vi "ziExample-Module-DAQ_Spectrum.vi"() -> ()   [LabVIEW 2009]
doc: "Control a Zurich instrument device via the LabOne Labview API. \nRequirements: Zurich Instruments MFLI, HF2 or UHFLI \nThis example shows how to start a spectrum modul and retrieve the Data.\n\n© Zurich Instruments AG, www.zhinst.com"
uses:
  <instrlib>/Zurich Instruments LabOne/Public/Data/ziTypeDoubleDataTS.ctl
  <instrlib>/Zurich Instruments LabOne/Public/Modules/ziTypeModResults.ctl
  <instrlib>/Zurich Instruments LabOne/Public/Data/ziTypePollType.ctl
  <instrlib>/Zurich Instruments LabOne/Public/Modules/ziTypeModGenericHeader.ctl
  <instrlib>/Zurich Instruments LabOne/Public/Modules/ziTypeModEnum.ctl
  <instrlib>/Zurich Instruments LabOne/Public/Modules/ziModSetValueDoubleArray.vi
  <instrlib>/Zurich Instruments LabOne/Public/Modules/ziModSetValueBinary.vi
  <instrlib>/Zurich Instruments LabOne/Public/Configure/ziSetValueDouble.vi
  <instrlib>/Zurich Instruments LabOne/Public/Modules/ziModGetNodeValueDouble.vi
  <instrlib>/Zurich Instruments LabOne/Public/Modules/ziModGetDoubleData.vi
  <instrlib>/Zurich Instruments LabOne/Zurich Instruments LabOne.lvlib
panel:
  out "Finished":bool
  out "Duration":dbl caption="Duration (s)"
  out "Progress (unity)":dbl(slide) step=1.10684602706915e-310 scale=0.0..100.0
  out "Filter":T1[](array[typedef])
  out "Header":T2
  out "Spectrum":T1[](array[typedef])
  in  "subscribepath":string="demods/0/sample.XiY.fft.abs.avg"
  in  "start_act":bool
  in  "stop":bool
  out "Error Out":errorcluster
  out "Power":bool
  out "SpectrumAbs":cluster{dbl[], "Value":dbl[]}[](graph)
  in  "refreshrate":dbl=5.0
  in  "frequencyspan":dbl=13000.0
  in  "Window":u16(ring) items=["Rectangular", "Hann", "Hamming", "Blackman Harris"]
  in  "Absolute":bool
  in  "specdens":bool caption="Spectral Density"
  in  "filtcomp":bool caption="Filter Compensation"
  in  "Address":string="DEV"
  out "Selected Device":string
  # "ziExample-Module-DAQ_Spectrum.vi\nRequirements: HF2LI, UHFLI or MFLI\nsee block diagram for VI description"
  # "Tested Devices:\n- HF2LI\n- UHFLI\n- MFLI"
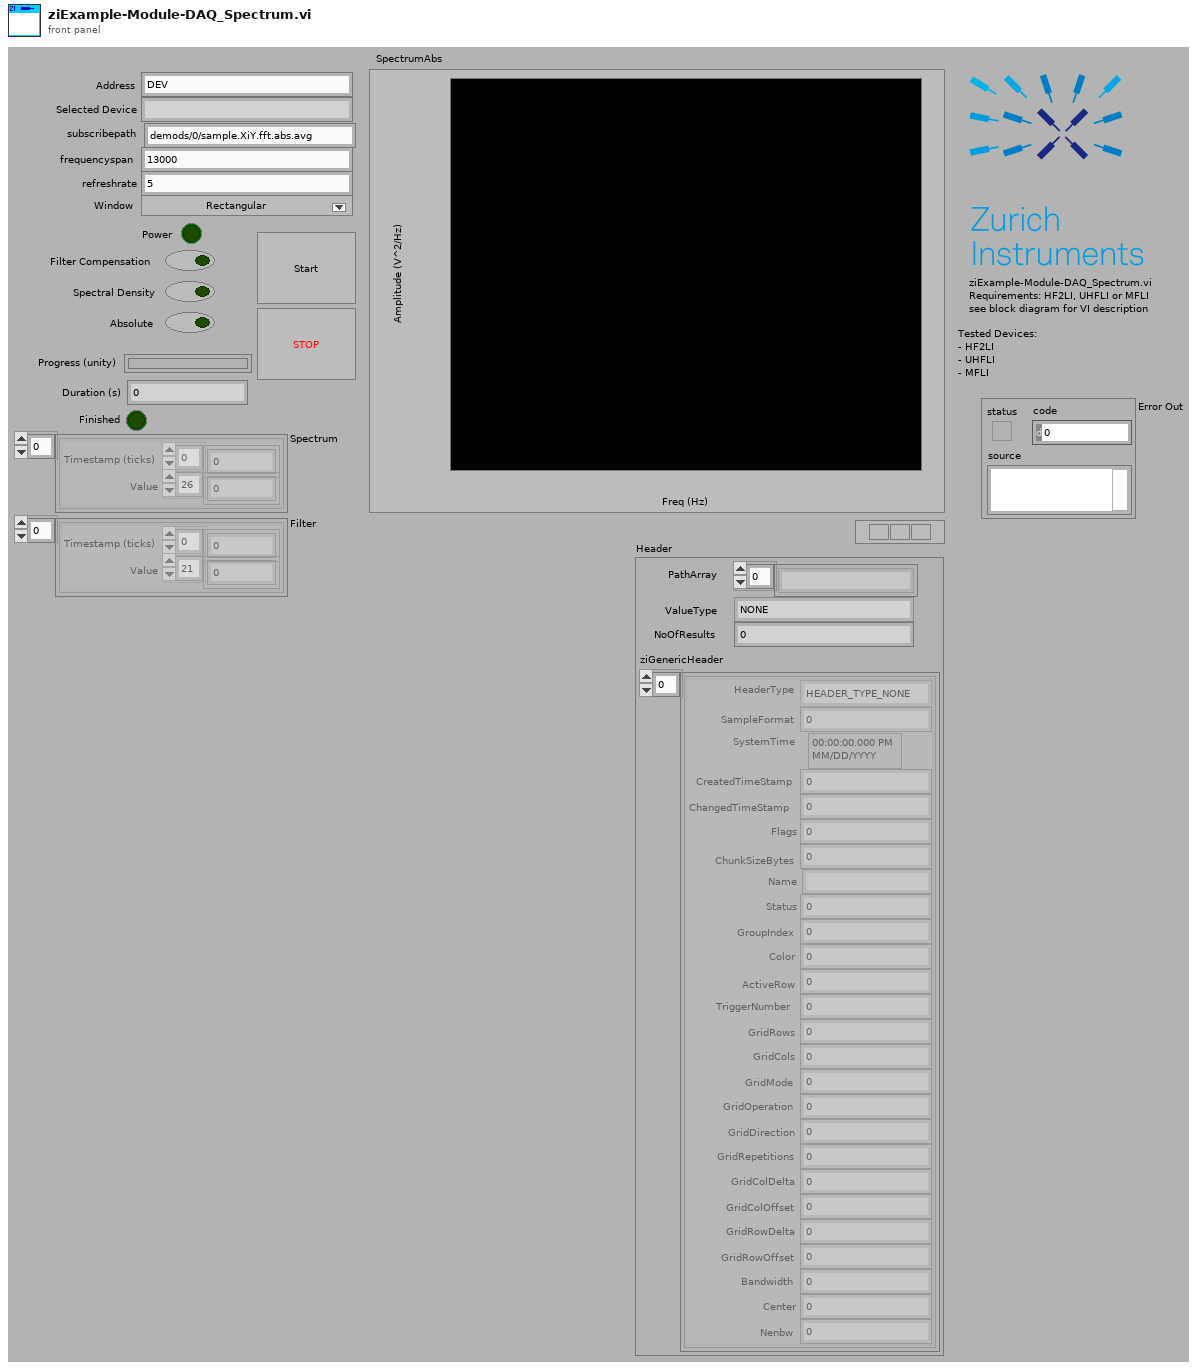
[diagram p1: front panel]
types:
  T1 = typedef "Zurich Instruments LabOne.lvlib/ziTypeDoubleDataTS.ctl" = cluster{"Timestamp (ticks)":u64[], "Value":dbl[]}
  T2 = typedef "Zurich Instruments LabOne.lvlib/ziTypeModResults.ctl" = cluster{"PathArray":string[], "ValueType":T3, "NoOfResults":u64, "ziGenericHeader":T4[]}
  T3 = typedef "Zurich Instruments LabOne.lvlib/ziTypePollType.ctl" = enum16{"NONE", "DOUBLE_DATA", "INTEGER_DATA", "DEMOD_SAMPLE", "SCOPE_WAVE_HF2", "AUXIN_SAMPLE", "DIO_SAMPLE", "BYTE_ARRAY", "PWA_WAVE", "9", "10", "11", "12", "13", "14", "15", "TREE_CHANGE_DEPRI", "17", "ERROR", "19", "20", "21", "22", "23", "24", "25", "26", "27", "28", "29", "30", "31", "DOUBLE_DATA_TS", "INTEGER_DATA_TS", "34", "SCOPE_WAVE", "SCOPE_WAVE_EX", "37", "BYTE_ARRAY_TS", "39", "40", "41", "42", "43", "44", "45", "CNT_DATA", "47", "TREE_CHANGE", "49", "50", "51", "52", "53", "54", "55", "56", "57", "58", "59", "60", "61", "62", "63", "SWEEPER_DATA", "SPECTRUM_DATA", "ADVISOR_DATA", "VECTOR_DATA", "IMP_DATA"}
  T4 = typedef "Zurich Instruments LabOne.lvlib/ziTypeModGenericHeader.ctl" = cluster{"HeaderType":enum8{"HEADER_TYPE_NONE", "HEADER_TYPE_SWTRIGGER", "HEADER_TYPE_SWEEPER"}, "SampleFormat":u8, "SystemTime":timestamp, "CreatedTimeStamp":u64, "ChangedTimeStamp":u64, "Flags":u32, "ChunkSizeBytes":u64, "Name":string, "Status":u32, "GroupIndex":u32, "Color":u32, "ActiveRow":u32, "TriggerNumber":u64, "GridRows":u32, "GridCols":u32, "GridMode":u32, "GridOperation":u32, "GridDirection":u32, "GridRepetitions":u32, "GridColDelta":dbl, "GridColOffset":dbl, "GridRowDelta":dbl, "GridRowOffset":dbl, "Bandwidth":dbl, "Center":dbl, "Nenbw":dbl}
  T5 = typedef "Zurich Instruments LabOne.lvlib/ziTypeModEnum.ctl" = u16
  T6 = typedef "Zurich Instruments LabOne.lvlib/ziTypeHandle.ctl" = cluster{"handleValid":bool, "Conn":u64, "Path Prefix":string, "Handle":u64, "Connected":bool, "Clockbase(s)":dbl}
  T7 = typedef "Zurich Instruments LabOne.lvlib/ziTypeModHandle.ctl" = cluster{"handleValid":bool, "Conn":u64, "ModHandle":u64, "moduleID":string, "Path Prefix":string}
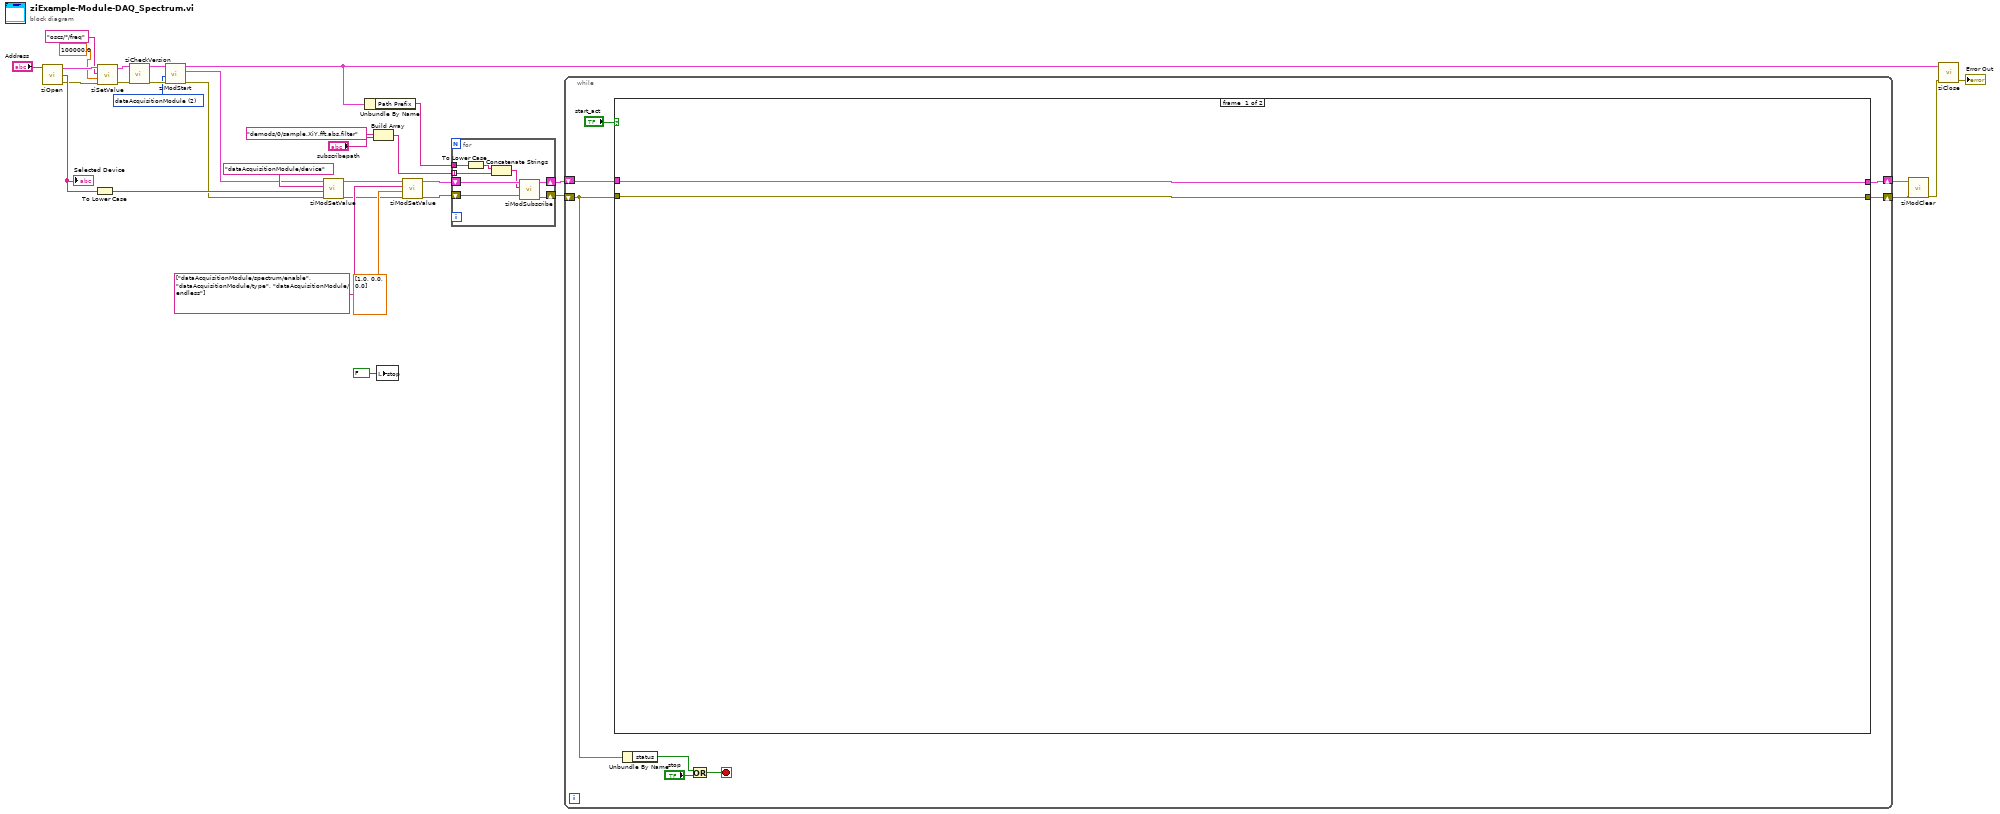
[diagram p0: block diagram]
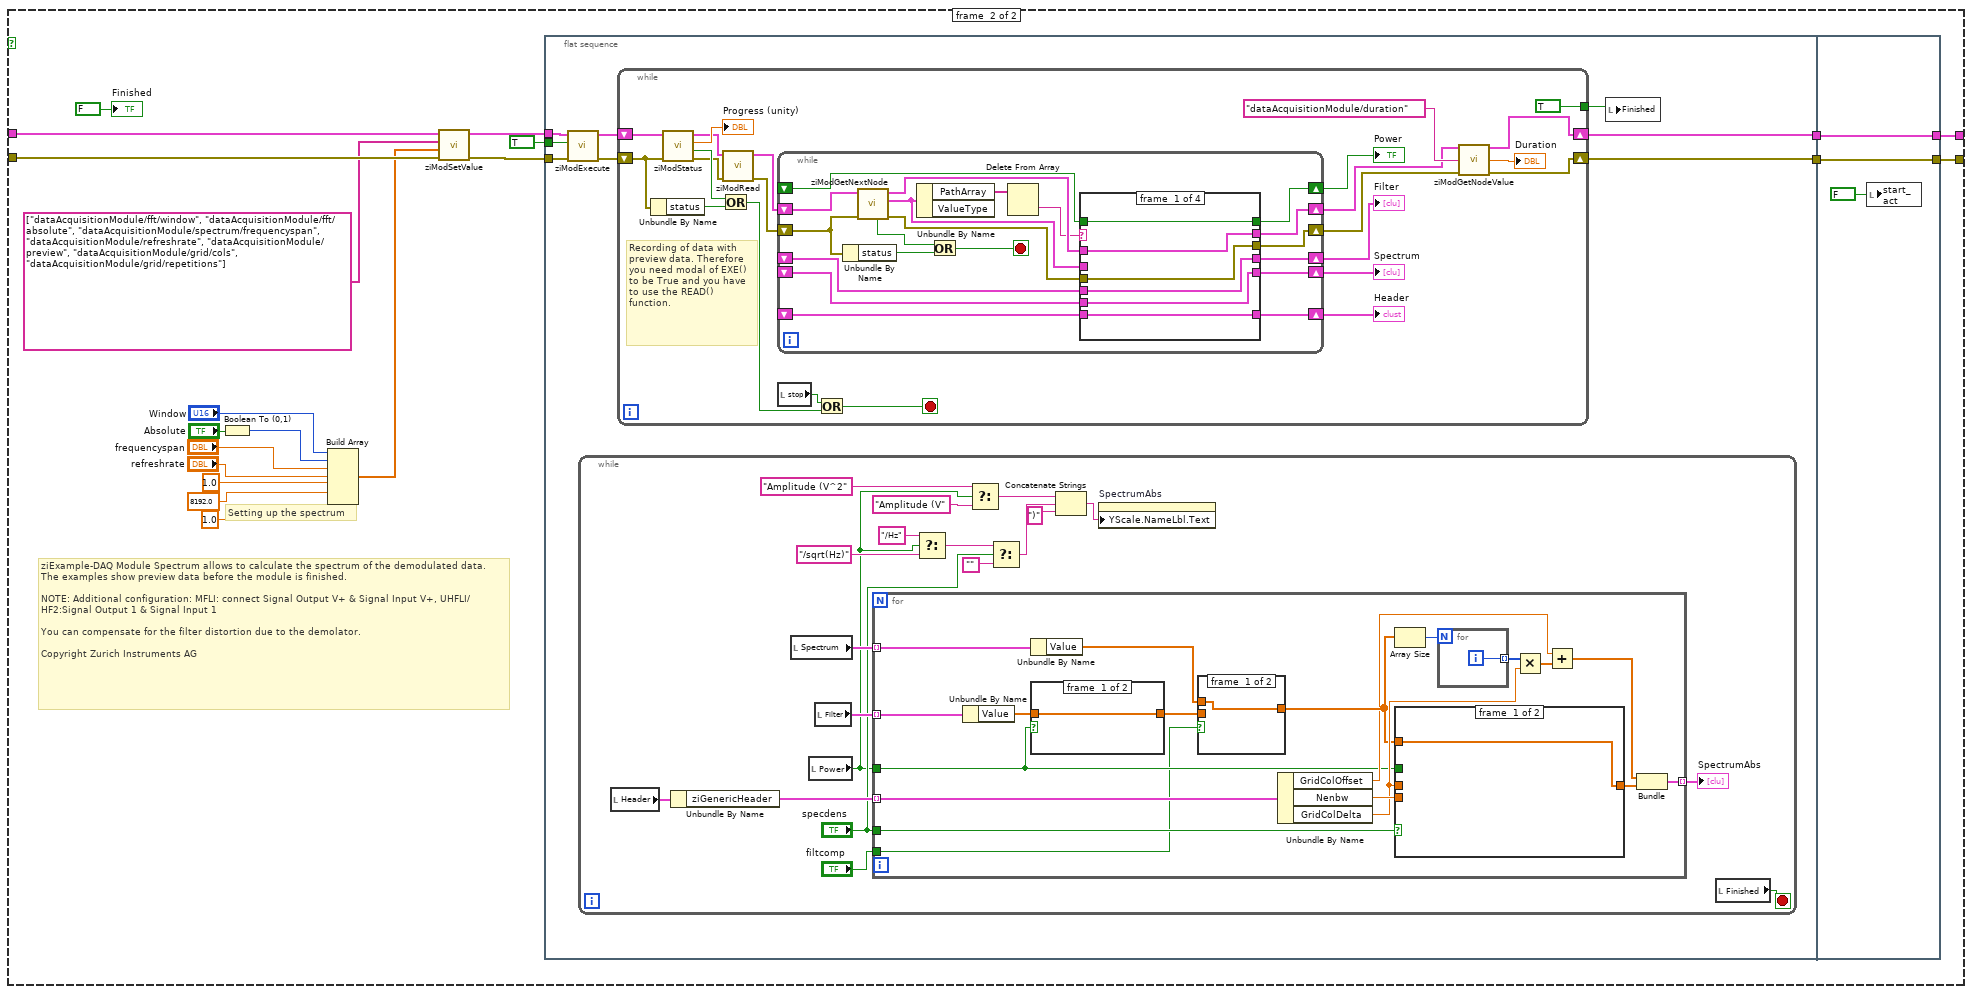
[diagram p2: hidden frame]
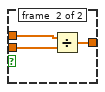
[diagram p3: hidden frame]
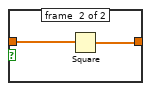
[diagram p4: hidden frame]
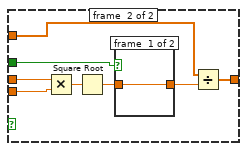
[diagram p5: hidden frame]
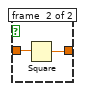
[diagram p6: hidden frame]
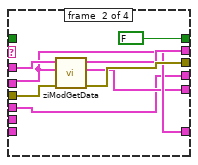
[diagram p7: hidden frame]
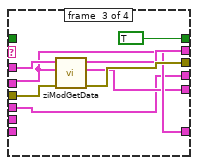
[diagram p8: hidden frame]
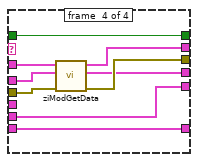
[diagram p9: hidden frame]
diagram:
  w8 = T5 2 items=["sweep", "scopeModule", "dataAcquisitionModule", "pidAdvisor", "awgModule", "impedanceModule", "multiDeviceSyncModule", "zoomFFT", "trigger", "deviceSettings", "record"] ("module Id")
  n1 = call <instrlib>:"ziOpen.vi"("Address"="Address") -> ("Error Out"=w11:errorcluster, "Selected Device"=w32:string, "HandleOut"=w12:T6)  [unwired: 3 in]
  "Selected Device" <- w32
  n2 = To Lower Case(string=w32) -> (all lower case string=w24:string)
  n3 = call-poly <instrlib>:"ziSetValue.vi"("Error In"=w11, "Value"=100000.0, "Path"="oscs/*/freq", "Handle In"=w12) -> ("Error Out"=w14:errorcluster, "Handle Out"=w13:T6)  [unwired: 1 in]
  n4 = call <instrlib>:"ziCheckVersion.vi"("Handle In"=w13, "Error In"=w14) -> ("Handle Out"=w27:T6, "Error Out"=w28:errorcluster)  [unwired: 11 in, 1 out]
  n5 = call <instrlib>:"ziModStart.vi"("Error In"=w28, "module Id"=w8, "Handle In"=w27) -> ("Error Out"=w22:errorcluster, "ModHandle Out"=w23:T7, "Handle Out"=w15:T6)  [unwired: 6 in]
  n6 = call-poly <instrlib>:"ziModSetValue.vi"("Error In"=w22, "Data"=w24, "Path"="dataAcquisitionModule/device" ("path"), "ModHandle In"=w23) -> ("Error Out"=w17:errorcluster, "ModHandle Out"=w18:T7)  [unwired: 6 in]
  n7 = Unbundle By Name(w15) -> ("Path Prefix"=w2:string)
  n8 = Build Array("demods/0/sample.XiY.fft.abs.filter", "subscribepath") -> (w1:string[])
  n9 = local write "stop"(FALSE ("Stop")) -> ()
  n10 = call-poly <instrlib>:"ziModSetValue.vi"("Error In"=w17, "Values"=dbl[] [1.0, 0.0, 0.0], "Paths"=string[] ["dataAcquisitionModule/spectrum/enable", "dataAcquisitionModule/type", "dataAcquisitionModule/endless"], "ModHandle In"=w18) -> ("Error Out"=w3:errorcluster, "ModHandle Out"=w16:T7)  [unwired: 6 in]
  n11 = for {
    shift-right: [w41] -> w21
    shift-left: w16 -> [w40]
    shift-right: [w34] -> w4
    shift-left: w3 -> [w35]
    tunnel: w2 -> [w37]
    tunnel: w1 -> [w36] mode=indexing
    n12 = To Lower Case(string=w37) -> (all lower case string=w38:string)
    n13 = Concatenate Strings(w38, w36) -> (w39:string)
    n14 = call <instrlib>:"ziModSubscribe.vi"("Error In"=w35, "Path"=w39, "ModHandle In"=w40) -> ("Error Out"=w34:errorcluster, "ModHandle Out"=w41:T7)  [unwired: 6 in]
  }
  n15 = while {
    shift-right: [w43] -> w26
    shift-left: w21 -> [w42]
    shift-right: [w49] -> w30
    shift-left: w4 -> [w45]
    stop <- w46 stop-if-true
    n16 = case shown="True" "start_act" {
      tunnel: w42 -> [w50 w71]
      tunnel: w45 -> [w51 w70]
      tunnel: [w50 w68] -> w43
      tunnel: [w51 w69] -> w49
      frame #0 {
      }
      frame #1 {
        # "Setting up the spectrum"
        # "ziExample-DAQ Module Spectrum allows to calculate the spectrum of the demodulated data.  The examples show preview data before the module is finished.\n \nNOTE: Additional configuration: MFLI: connect Signal Output V+ & Signal Input V+, UHFLI/HF2:Signal Output 1 & Signal Input 1\n\nYou can compensate for the filter distortion due to the demolator.\n\nCopyright Zurich Instruments AG"
        n17 = Boolean To (0,1)(Boolean="Absolute") -> (0, 1=w63:i16)
        n18 = Build Array("Window", w63, "frequencyspan", "refreshrate", 1.0 ("element"), 8192.0 ("element"), 1.0 ("element")) -> (w64:dbl[])
        n19 = call-poly <instrlib>:"ziModSetValue.vi"("Error In"=w70, "Values"=w64, "Paths"=string[] ["dataAcquisitionModule/fft/window", "dataAcquisitionModule/fft/absolute", "dataAcquisitionModule/spectrum/frequencyspan", "dataAcquisitionModule/refreshrate", "dataAcquisitionModule/preview", "dataAcquisitionModule/grid/cols", "dataAcquisitionModule/grid/repetitions"], "ModHandle In"=w71) -> ("Error Out"=w55:errorcluster, "ModHandle Out"=w56:T7)  [unwired: 6 in]
        n20 = flat-sequence {
          tunnel: TRUE ("Modal") -> [w77]
          tunnel: w56 -> [w76]
          tunnel: w55 -> [w75]
          tunnel: [w79] -> w58
          tunnel: [w78] -> w57
          tunnel: [w213] -> w68
          tunnel: [w214] -> w69
          tunnel: w58 -> [w214]
          tunnel: w57 -> [w213]
          frame #0 {
            n21 = call <instrlib>:"ziModExecute.vi"("Error In"=w75, "Modal (F)"=w77, "ziModHandle In"=w76) -> ("Error Out"=w74:errorcluster, "ziModHandle Out"=w73:T7)  [unwired: 5 in, 1 out]
            n22 = while {
              stop <- w83 stop-if-true
              n23 = local read "Header"() -> (w86:T2)
              n24 = Unbundle By Name(w86) -> ("ziGenericHeader"=w88:T4[])
              n25 = local read "Spectrum"() -> (w87:T1[])
              n26 = local read "Power"() -> (w81:bool)
              n27 = local read "Filter"() -> (w85:T1[])
              n28 = for {
                tunnel: w87 -> [w117] mode=indexing
                tunnel: w85 -> [w116] mode=indexing
                tunnel: [w109] -> w84 mode=indexing
                tunnel: w88 -> [w114] mode=indexing
                tunnel: w81 -> [w100]
                tunnel: "specdens" -> [w103]
                tunnel: "filtcomp" -> [w99]
                n29 = Unbundle By Name(w116) -> ("Value"=w102:dbl[])
                n30 = Unbundle By Name(w117) -> ("Value"=w105:dbl[])
                n31 = case shown="True" w100 {
                  tunnel: w102 -> [w122 w124]
                  tunnel: [w122 w123] -> w101
                  frame #0 {
                  }
                  frame #1 {
                    n32 = Square(x=w124) -> (x^2=w123:dbl[])
                  }
                }
                n33 = case shown="False" w99 {
                  tunnel: [w118 w121] -> w107
                  tunnel: w105 -> [w118 w120]
                  tunnel: w101 -> [_ w119]
                  frame #0 {
                  }
                  frame #1 {
                    n34 = Divide(x=w120, y=w119) -> (x/y=w121:dbl[])
                  }
                }
                n35 = Unbundle By Name(w114) -> ("GridColOffset"=w106:dbl, "Nenbw"=w113:dbl, "GridColDelta"=w108:dbl)
                n36 = Array Size(array=w107) -> (size(s)=w115:i32)
                n37 = case shown="True" w103 {
                  tunnel: w107 -> [w126 w133]
                  tunnel: [w126 w132] -> w104
                  tunnel: w108 -> [_ w131]
                  tunnel: w113 -> [_ w130]
                  tunnel: w100 -> [_ w127]
                  frame #0 {
                  }
                  frame #1 {
                    n38 = Multiply(x=w131, y=w130) -> (x*y=w134:dbl)
                    n39 = Square Root(x=w134) -> (sqrt(x)=w129:dbl)
                    n40 = case shown="True" w127 {
                      tunnel: w129 -> [w135 w137]
                      tunnel: [w135 w136] -> w128
                      frame #0 {
                      }
                      frame #1 {
                        n41 = Square(x=w137) -> (x^2=w136:dbl)
                      }
                    }
                    n42 = Divide(x=w133, y=w128) -> (x/y=w132:dbl[])
                  }
                }
                n43 = for {
                  N: w115 -> [_]
                  tunnel: [w125] -> w111 mode=indexing
                  i -> [w125]
                }
                n44 = Multiply(x=w111, y=w108) -> (x*y=w112:dbl[])
                n45 = Add(x=w106, y=w112) -> (x+y=w110:dbl[])
                n46 = Bundle(w110, "Value"=w104) -> (w109:cluster{dbl[], "Value":dbl[]})  [unwired: 1 in]
              }
              "SpectrumAbs" <- w84
              n47 = Select(t="/Hz", s=w81, f="/sqrt(Hz)") -> (s? t:f=w89:string)
              n48 = Select(t="Amplitude (V^2", s=w81, f="Amplitude (V") -> (s? t:f=w92:string)
              n49 = Select(t=w89, s="specdens", f="") -> (s? t:f=w97:string)
              n50 = Concatenate Strings(w92, w97, ")") -> (w96:string)
              n51 = property on="SpectrumAbs" class="XYGraph (strict)"("YScale.NameLbl.Text"=w96) -> ()  [unwired: 2 in, 2 out]
              n52 = local read "Finished"() -> (w83:bool)
            }
            n53 = while {
              shift-right: [w149] -> w79
              shift-left: w74 -> [w145]
              shift-right: [w154] -> w78
              shift-left: w73 -> [w148]
              tunnel: [TRUE] -> w72
              stop <- w150 stop-if-true
              # "Recording of data with preview data. Therefore you need modal of EXE() to be True and you have to use the READ() function."
              n54 = Unbundle By Name(w145) -> ("status"=w160:bool)
              n55 = call <instrlib>:"ziModStatus.vi"("Error In"=w145, "ModHandle IN"=w148) -> ("Error Out"=w146:errorcluster, "Finished?"=w153:bool, "Progress (unity)"=→"Progress (unity)":dbl, "ModHandle Out"=w147:T7)  [unwired: 5 in]
              n56 = Or(x=w153, y=w160) -> (x .or. y?=w151:bool)
              n57 = call <instrlib>:"ziModRead.vi"("error in"=w146, "ziModHandle In"=w147) -> ("error out"=w158:errorcluster, "ziModHandle Out"=w157:T7)  [unwired: 8 in]
              n58 = while {
                shift-right: [w170] -> w143
                shift-left: w157 -> [w169]
                shift-right: [w171] -> w144
                shift-left: w158 -> [w178]
                shift-right: [w168] -> w138
                shift-left: _ -> [w167]
                shift-right: [w166] -> w139
                shift-left: _ -> [w165]
                shift-right: [w164] -> w140
                shift-left: _ -> [w163]
                shift-right: [w162] -> w141
                shift-left: _ -> [w161]
                stop <- w177 stop-if-true
                n59 = Unbundle By Name(w178) -> ("status"=w172:bool)
                n60 = call <instrlib>:"ziModGetNextNode.vi"("Error In"=w178, "ModHandle In"=w169) -> ("Error Out"=w179:errorcluster, "ModResults"=w174:T2, "ModHandle Out"=w180:T7, "NoData"=w173:bool)  [unwired: 6 in]
                n61 = Unbundle By Name(w174) -> ("PathArray"=w176:string[])  [unwired: 1 out]
                n62 = Or(x=w173, y=w172) -> (x .or. y?=w177:bool)
                n63 = Delete From Array(array=w176) -> (deleted portion=w175:string)  [unwired: 2 in, 1 out]
                n64 = case shown="Default" w175 {
                  tunnel: w180 -> [w186 w194 w202 w210]
                  tunnel: w174 -> [_ w190 w198 w211]
                  tunnel: w179 -> [w185 w193 w201 w209]
                  tunnel: [w185 w192 w200 w208] -> w171
                  tunnel: [w186 w191 w199 w207] -> w170
                  tunnel: [w182 w190 w198 w204] -> w164
                  tunnel: [w183 w189 w197 w205] -> w166
                  tunnel: [w184 w188 w196 w206] -> w168
                  tunnel: w167 -> [w184 w188 w196 _]
                  tunnel: w165 -> [w183 _ _ w205]
                  tunnel: w163 -> [w182 _ _ w204]
                  tunnel: [w181 FALSE TRUE w203] -> w162
                  tunnel: w161 -> [w181 _ _ w203]
                  frame #0 {
                  }
                  frame #1 {
                    n65 = call-poly <instrlib>:"ziModGetData.vi"("Error In"=w193, "ModResults"=w190, "ModHandle In"=w194) -> ("Error Out"=w192:errorcluster, "DoubleSample"=w189:T1[], "ModHandle Out"=w191:T7)  [unwired: 4 in, 2 out]
                  }
                  frame #2 {
                    n66 = call-poly <instrlib>:"ziModGetData.vi"("Error In"=w201, "ModResults"=w198, "ModHandle In"=w202) -> ("Error Out"=w200:errorcluster, "DoubleSample"=w197:T1[], "ModHandle Out"=w199:T7)  [unwired: 4 in, 2 out]
                  }
                  frame #3 {
                    n67 = call-poly <instrlib>:"ziModGetData.vi"("Error In"=w209, "ModResults"=w211, "ModHandle In"=w210) -> ("Error Out"=w208:errorcluster, "DoubleSample"=w206:T1[], "ModHandle Out"=w207:T7)  [unwired: 4 in, 2 out]
                  }
                }
              }
              "Filter" <- w138
              "Spectrum" <- w139
              "Header" <- w140
              "Power" <- w141
              n68 = local read "stop"() -> (w152:bool)
              n69 = Or(x=w152, y=w151) -> (x .or. y?=w150:bool)
              n70 = call-poly <instrlib>:"ziModGetNodeValue.vi"("ModHandle In"=w143, "Path"="dataAcquisitionModule/duration", "error in"=w144) -> ("ModHandle Out"=w154:T7, "Value"=→"Duration":dbl, "error out"=w149:errorcluster)  [unwired: 10 in]
            }
            n71 = local write "Finished"(w72) -> ()
          }
          frame #1 {
            n72 = local write "start_act"(FALSE ("start_act")) -> ()
          }
        }
        "Finished" <- FALSE
      }
    }
    n73 = Unbundle By Name(w45) -> ("status"=w47:bool)
    n74 = Or(x=w47, y="stop") -> (x .or. y?=w46:bool)
  }
  n75 = call <instrlib>:"ziModClear.vi"("Error In"=w30, "ziModHandle In"=w26) -> ("Error Out"=w33:errorcluster)  [unwired: 7 in, 1 out]
  n76 = call <instrlib>:"ziClose.vi"("Error In"=w33, "Handle In"=w15) -> ("Error Out"=→"Error Out":errorcluster)  [unwired: 2 in, 1 out]
